vi "push.vi"(8 "error in (no error)":errorcluster, 10 "Mission.lvclass":refnum<class "Mission.lvclass">, 11 "MissionQueue in":refnum<class "MissionQueue.lvclass">) -> (0 "error out":errorcluster, 3 "MissionQueue out":refnum<class "MissionQueue.lvclass">)   [LabVIEW 2011]
doc: "Add a new Mission to the MissionQueue."
uses:
  MissionQueue.lvclass
  Mission/Mission.lvclass
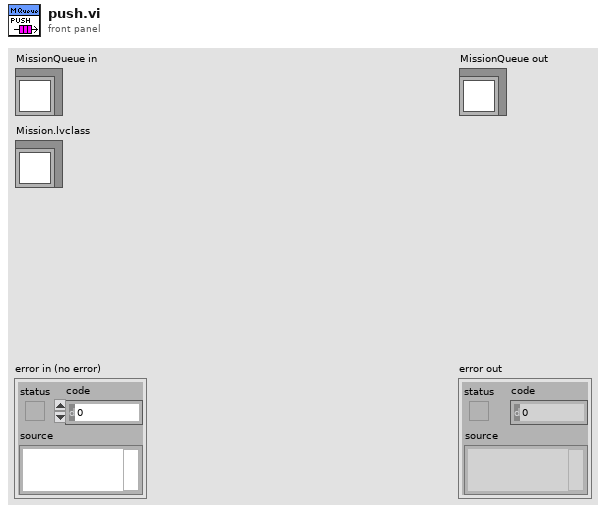
[diagram p1: front panel]
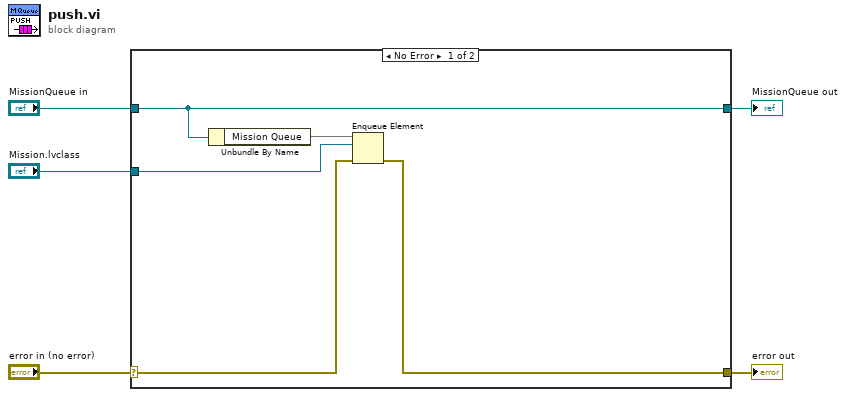
[diagram p0: block diagram]
diagram:
  n1 = case shown="No Error" "error in (no error)" {
    selector: "error in (no error)" -> [w8 w12]
    tunnel: [w6 w12] -> w4
    tunnel: [w7 w11] -> w2
    tunnel: "MissionQueue in" -> [w7 w11]
    tunnel: "Mission.lvclass" -> [w9 _]
    frame No Error {
      n2 = Unbundle By Name(w7) -> ("Mission Queue"=w10)
      n3 = Enqueue Element(queue=w10, element=w9, error in (no error)=w8) -> (error out=w6:errorcluster)  [unwired: 1 in, 2 out]
    }
    frame Error {
    }
  }
  "error out" <- w4
  "MissionQueue out" <- w2
